vi "Global variables.vi"() -> ()   [LabVIEW 2017]
panel:
  in  "DAC manager step":u8
  in  "hinge cluster":T1 {"transition" items=["Step", "Ramp", "Exp", "Bin"]}
  in  "DAC manager channel":u8
  in  "DAC manager set values":bool
  in  "DAC manager break+update+loop":bool
  out "Evasp calc'd time":dbl
  out "Repeat end ptr":i32
  out "Repetition count":i32
  out "Repeat enabled":bool
  out "Repeat stack":string
  out "Total repetition":i32
  out "Variable loop enabled":bool
  out "Loop total":i32
  out "Loop cnt":i32
  out "indices":i32[](array[numeric])
  in  "value table":dbl[][](array[numeric])
  in  "Variables defined":string[](array[string])
  # "time (ms)"
  # "voltage (V)"
  # "transition"
  # "tau (ms)"
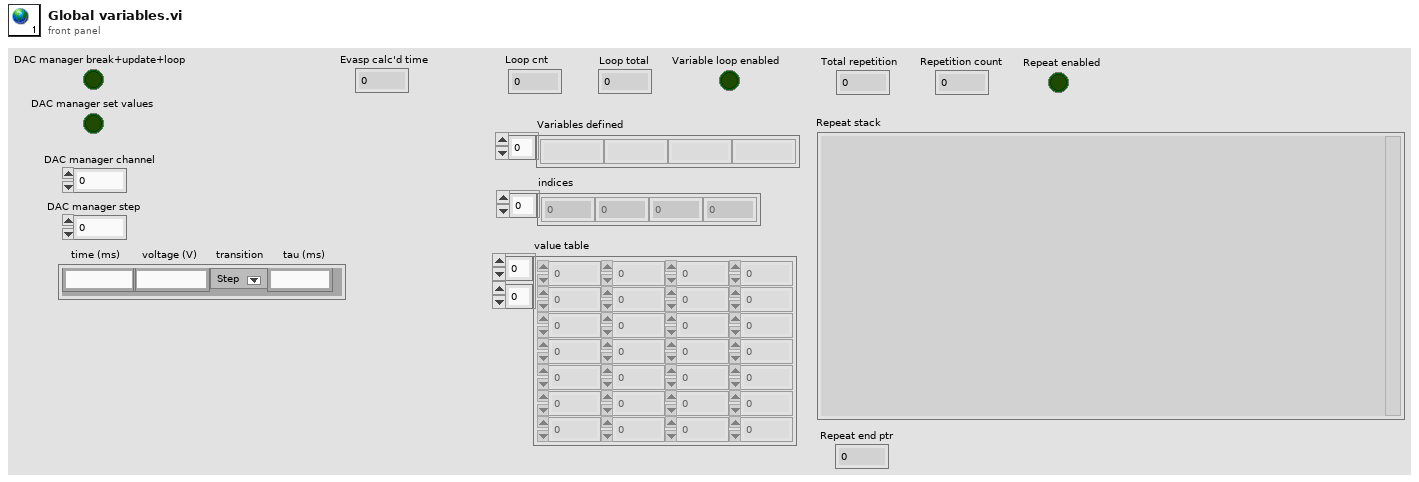
[diagram p1: front panel]
types:
  T1 = cluster{"time (ms)":string, "voltage (V)":string, "transition":u16, "tau":string}
diagram:
